vi "GetAllFurniture.vi"(8 "error in (no error)":errorcluster, 11 "Room in":refnum<class "Room.lvclass">) -> (0 "error out":errorcluster, 2 "Furniture":refnum<class "Furniture.lvclass">[](array[class]), 3 "Room out":refnum<class "Room.lvclass">)   [LabVIEW 2019, in "Room.lvclass"]
uses:
  Room.lvclass
  Furniture.lvclass
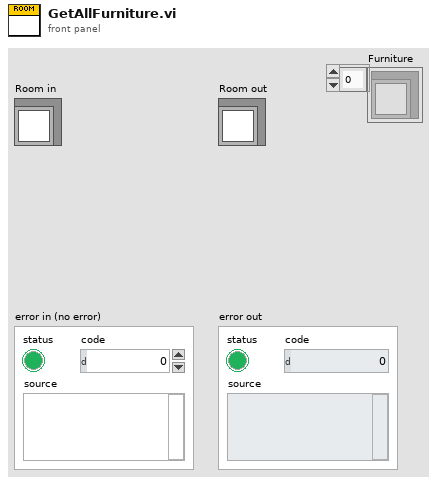
[diagram p1: front panel]
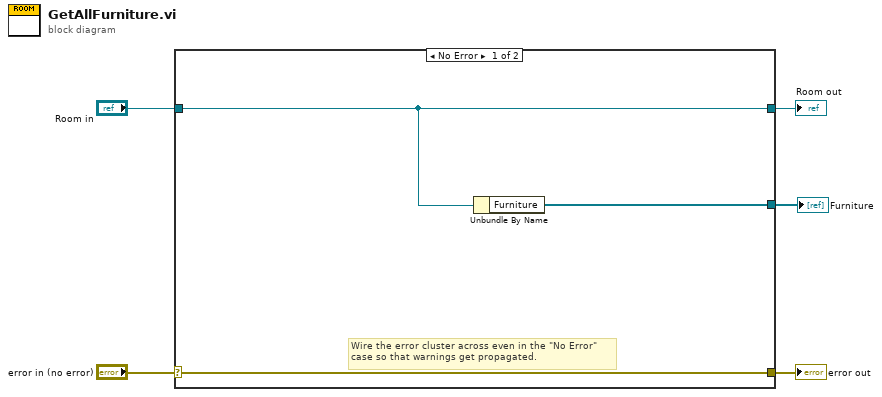
[diagram p0: block diagram]
diagram:
  n1 = case shown="No Error" "error in (no error)" {
    selector: "error in (no error)" -> [w8 w10]
    tunnel: [w8 w10] -> w2
    tunnel: [w7 w9] -> w4
    tunnel: "Room in" -> [w7 w9]
    tunnel: [w6 _] -> w1
    frame No Error {
      # "Wire the error cluster across even in the \"No Error\"\ncase so that warnings get propagated."
      n2 = Unbundle By Name(w7) -> ("Furniture"=w6:refnum<class "Furniture.lvclass">[])
    }
    frame Error {
    }
  }
  "Room out" <- w4
  "error out" <- w2
  "Furniture" <- w1
